vi "Barcode print.vi"(9 "Str Refnum":refnum<vi>, 10 "Printer":enum16{"RS232  PrintOut", "USB Print Out"}(ring), 11 "Boolean 3":bool) -> (0 "error out":errorcluster)   [LabVIEW 2015]
uses:
  <vilib>/Instr/_visa.llb/VISA Configure Serial Port (Instr).vi
panel:
  out "send on  barcode printer 2":string="﻿\u0010CT~~CD,~CC^~CT~\n^XA~TA000~JSN^LT0^MNW^MTT^PON^PMN^LH0,0^JMA^PR3,3~SD22^JUS^LRN^CI0^XZ\n^XA\n^MMT\n^PW1200\n^LL0300\n^LS0\n^FT44,48^AAN,54,20^FH\\^FDAUTHENTIC ENGINEERS^FS\n^BY4,3,139^FT61,196^BCN,,Y,N\n^FD>;050620151983^FS\n^PQ1,0,1,Y^XZ\n"
  out "send on  barcode printer":string="﻿\u0010CT~~CD,~CC^~CT~\n^XA~TA000~JSN^LT0^MNW^MTT^PON^PMN^LH0,0^JMA^PR3,3~SD22^JUS^LRN^CI0^XZ\n^XA\n^MMT\n^PW1200\n^LL0300\n^LS0\n^FT44,48^AAN,54,20^FH\\^FDAUTHENTIC ENGINEERS^FS\n^BY4,3,139^FT61,196^BCN,,Y,N\n^FD>;050620151983^FS\n^PQ1,0,1,Y^XZ\n"
  out "error out 4":errorcluster
  out "error out 3":errorcluster
  out "error out 2":errorcluster
  out "Serial no":string
  # "ft6,84\n6,76\n6,70\nft203,103\nft203,100\n203,98"
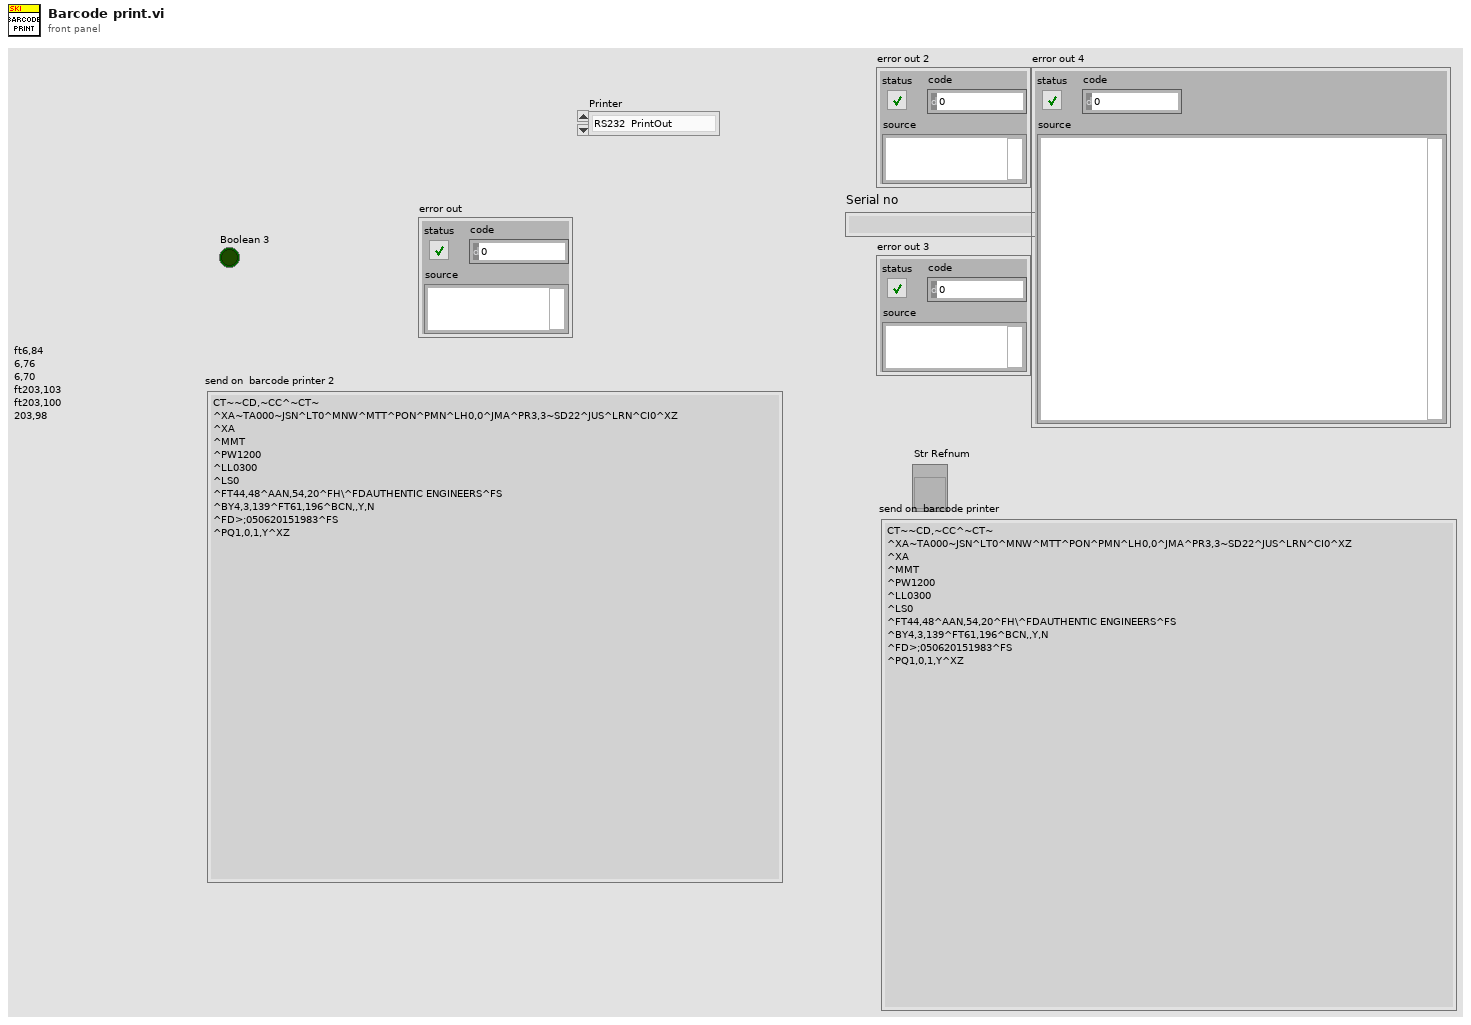
[diagram p1: front panel]
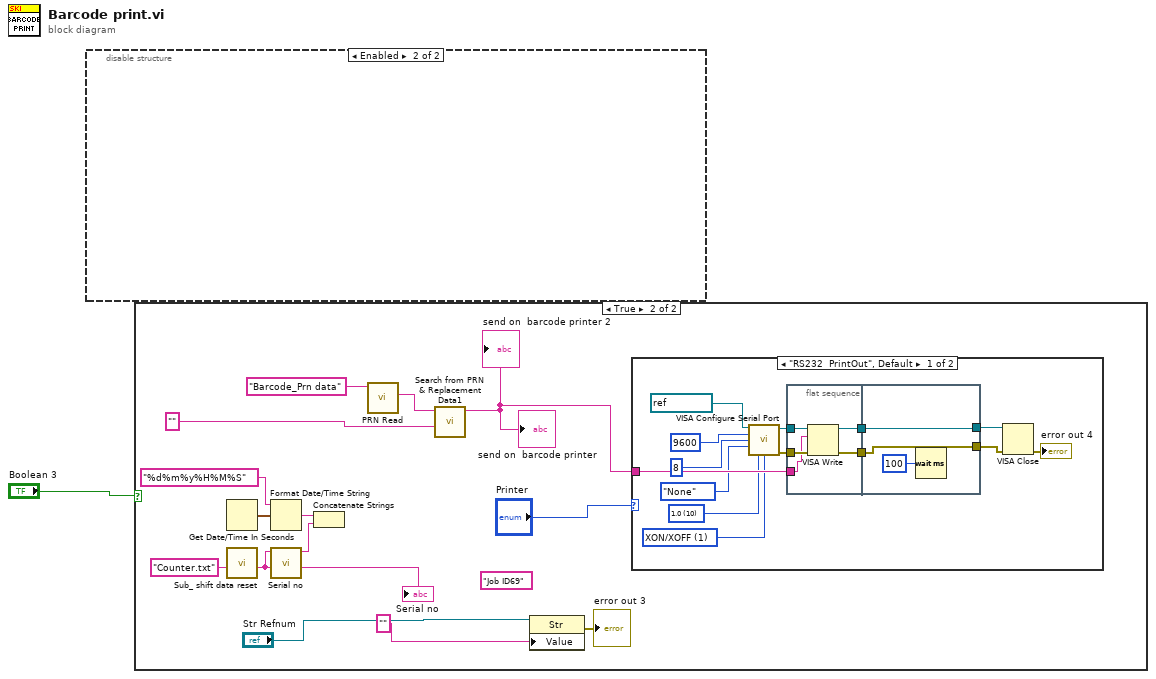
[diagram p0: block diagram]
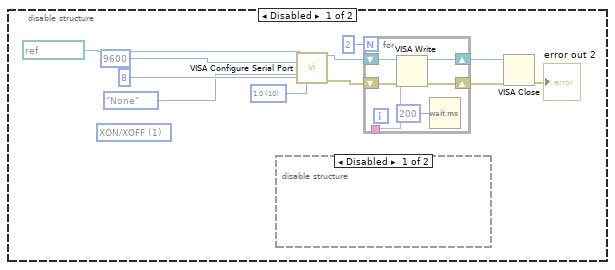
[diagram p2: hidden frame]
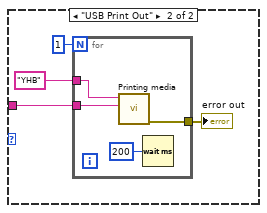
[diagram p5: hidden frame]
diagram:
  n1 = disable-structure shown="Enabled" {
    frame Disabled {
      (unwired) u16 1 items=["None", "XON/XOFF", "RTS/CTS", "XON/XOFF & RTS/CTS", "DTR/DSR", "XON/XOFF & DTR/DSR"] ("flow control (0:none)")
      w5 = u16 10 items=["1.0"=10, "1.5"=15, "2.0"=20] ("stop bits (10: 1 bit)")
      n2 = disable-structure shown="Disabled" {
        frame Disabled {
        }
        frame Enabled {
        }
      }
      n3 = call-poly "VISA Configure Serial Port"("VISA resource name"=refnum<visa-resource-name> "COM1", "baud rate (9600)"=u32 9600, "data bits (8)"=u16 8, "parity (0:none)"=enum16{"None", "Odd", "Even", "Mark", "Space"}."None", "stop bits (10: 1 bit)"=w5) -> ("VISA resource name out"=w13:refnum<visa-resource-name>, "error out"=w12:errorcluster)  [unwired: 9 in]
      n4 = for {
        N: 2 -> [_]
        tunnel: [w15] -> w3
        shift-right: [w17] -> w11
        shift-left: w13 -> [w19]
        shift-right: [w16] -> w10
        shift-left: w12 -> [w18]
        n5 = VISA Write(VISA resource name=w19, write buffer=w15, error in (no error)=w18) -> (VISA resource name out=w17:refnum<visa-resource-name>, error out=w16:errorcluster)  [unwired: 1 out]
        n6 = Wait (ms)(milliseconds to wait=u32 200) -> ()  [unwired: 1 out]
      }
      n7 = VISA Close(VISA resource name=w11, error in (no error)=w10) -> (error out=→"error out 2":errorcluster)
    }
    frame Enabled {
    }
  }
  n8 = case shown="True" "Boolean 3" {
    frame False {
    }
    frame True {
      (unwired) "Job ID69" ("printer name")
      n9 = Get Date/Time In Seconds() -> (seconds since 1Jan1904=w32:timestamp)
      n10 = call "Sub_ shift data reset.vi"("Serial no"="Counter.txt") -> ("Serial no"=w29:string)  [unwired: 8 in, 1 out]
      "Serial no" <- w29
      n11 = Format Date/Time String(time format string (%c)="%d%m%y%H%M%S", seconds (now)=w32) -> (date/time string=w31:string)  [unwired: 1 in]
      n12 = call "Serial no.vi"("Serial no"=w29) -> ("String"=w30:string)  [unwired: 10 in]
      n13 = Concatenate Strings(w31, w30) -> ()  [unwired: 1 out]
      n14 = call "PRN Read.vi"("prn"="Barcode_Prn data") -> ("Read Prn"=w26:string)  [unwired: 9 in, 1 out]
      n15 = call "Search from PRN  & Replacement Data1.vi"("PRN  Call File"=w26, "Model"="") -> ("PRN out"=w22:string)  [unwired: 7 in, 1 out]
      "send on  barcode printer" <- w22
      "send on  barcode printer 2" <- w22
      n16 = property class="Str"(reference="Str Refnum", "Value"="") -> (error out=→"error out 3":errorcluster)  [unwired: 1 in, 1 out]
      n17 = case shown="\"RS232  PrintOut\", Default" "Printer" {
        tunnel: w22 -> [w39 w59]
        frame "RS232  PrintOut", Default {
          w34 = u16 1 items=["None", "XON/XOFF", "RTS/CTS", "XON/XOFF & RTS/CTS", "DTR/DSR", "XON/XOFF & DTR/DSR"] ("flow control (0:none)")
          w35 = u16 10 items=["1.0"=10, "1.5"=15, "2.0"=20] ("stop bits (10: 1 bit)")
          n18 = call-poly "VISA Configure Serial Port"("VISA resource name"=refnum<visa-resource-name> "COM3", "baud rate (9600)"=u32 9600, "data bits (8)"=u16 8, "parity (0:none)"=enum16{"None", "Odd", "Even", "Mark", "Space"}."None", "stop bits (10: 1 bit)"=w35, "flow control (0:none)"=w34) -> ("VISA resource name out"=w46:refnum<visa-resource-name>, "error out"=w45:errorcluster)  [unwired: 3 in, 5 out]
          n19 = flat-sequence {
            tunnel: w46 -> [w52]
            tunnel: w45 -> [w51]
            tunnel: [w50] -> w43
            tunnel: [w49] -> w41
            tunnel: w39 -> [w48]
            tunnel: w43 -> [w55]
            tunnel: [w55] -> w42
            tunnel: w41 -> [w54]
            tunnel: [w54] -> w40
            frame #0 {
              n20 = VISA Write(VISA resource name=w52, write buffer=w48, error in (no error)=w51) -> (VISA resource name out=w50:refnum<visa-resource-name>, error out=w49:errorcluster)  [unwired: 1 out]
            }
            frame #1 {
              n21 = Wait (ms)(milliseconds to wait=u32 100) -> ()  [unwired: 1 out]
            }
          }
          n22 = VISA Close(VISA resource name=w42, error in (no error)=w40) -> (error out=→"error out 4":errorcluster)
        }
        frame "USB Print Out" {
          n23 = for {
            N: 1 -> [_]
            tunnel: w59 -> [w63]
            tunnel: "YHB" ("printer name") -> [w61]
            tunnel: [w60] -> w57
            n24 = call "Printing media.vi"("send on  barcode printer"=w63, "printer name"=w61) -> ("error out"=w60:errorcluster)  [unwired: 9 in]
            n25 = Wait (ms)(milliseconds to wait=u32 200) -> ()  [unwired: 1 out]
          }
          "error out" <- w57
        }
      }
    }
  }
